vi "PythonNode_testforloopcopy2.vi"() -> ()   [LabVIEW 2023]
doc: "This example demonstrates how to call a Python function and pass doubles as arguments. It uses a python function to compute the sum of two doubles."
uses:
  <vilib>/Utility/sysdir.llb/System Directory Type.ctl
  <vilib>/Utility/file.llb/Write Delimited Spreadsheet (string).vi
panel:
  out "Image":T1(plugin-control)
  out "Waveform Graph":dbl[](graph)
  out "possibility(%)":dbl format="%#_13g"
  out "ready?":string
  out "error out":errorcluster
  in  "error in (no error)":errorcluster
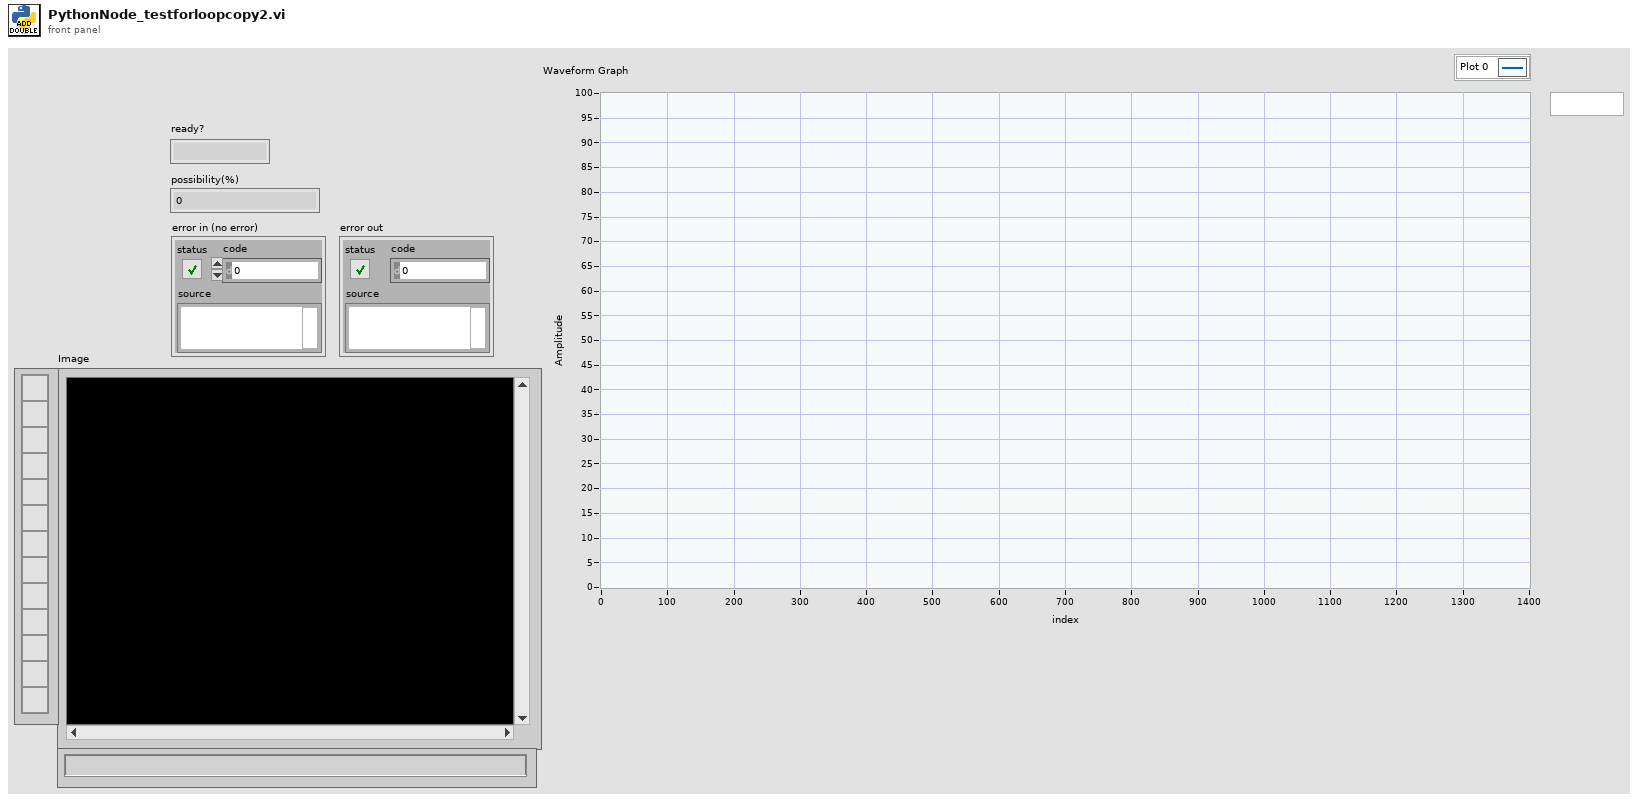
[diagram p1: front panel]
types:
  T1 = typedef "IMAQ Image.ctl" = refnum<image>
  T2 = typedef "System Directory Type.ctl" = i32
  T3 = typedef "Image Type" = u32
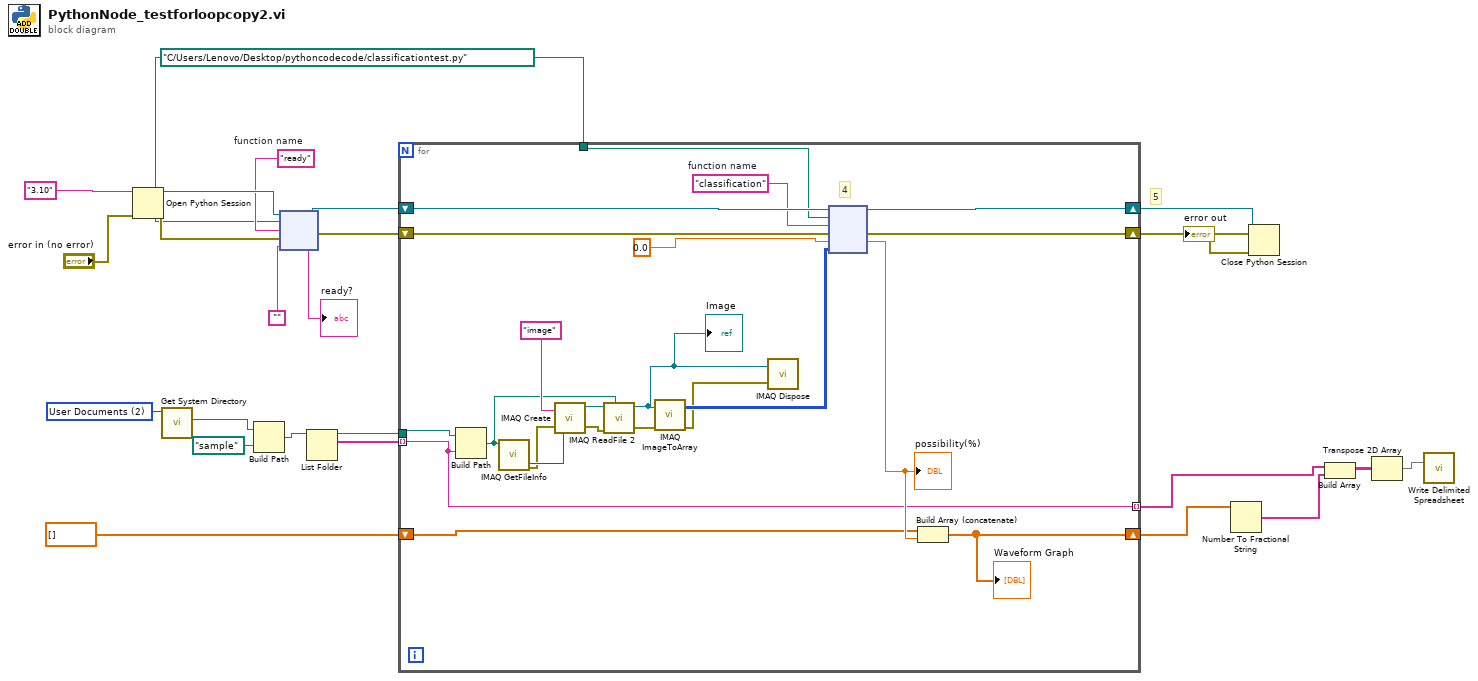
[diagram p0: block diagram]
diagram:
  w12 = T2 2 items=["User Home"=0, "User Desktop"=1, "User Documents"=2, "User Application Data"=3, "User Preferences"=4, "User Temporary"=5, "Public Documents"=6, "Public Application Data"=7, "Public Preferences"=8, "Public Cache"=13, "System Core Libraries"=9, "System Installed Libraries"=10, "Application Files"=11, "Boot Volume Root"=12] ("system directory type")
  w13 = path "C:/Users/Lenovo/Desktop/pythoncodecode/classificationtest.py" ("python file path")
  w21 = "ready"  # function name
  # "5"
  n1 = Open Python Session(python version="3.10", 3:"error in (no error)") -> (session out=w23:refnum<k35>, error out=w22:errorcluster)  [unwired: 1 in]
  n2 = call <vilib>:"Get System Directory.vi"("system directory type"=w12) -> ("system directory"=w11:path)  [unwired: 10 in]
  n3 = Build Path(base path=w11, name or relative path=path "sample") -> (appended path=w9:path)
  n4 = node(w23, w13, w21, w22, "") -> (w19:refnum<k35>, w18:errorcluster, →"ready?":string)  [unwired: 2 out]
  n5 = List Folder(path=w9) -> (path out=w7:path, filenames=w8:string[])  [unwired: 3 in, 2 out]
  n6 = for {
    tunnel: w13 -> [w43]
    shift-right: [w45] -> w17
    shift-left: w19 -> [w47]
    shift-right: [w44] -> w16
    shift-left: w18 -> [w46]
    tunnel: w8 -> [w27] mode=indexing
    tunnel: w7 -> [w36]
    shift-right: [w32] -> w5
    shift-left: dbl[] [] -> [w33]
    tunnel: [w27] -> w4 mode=indexing
    w42 = "classification"  # function name
    # "4"
    n7 = Build Path(base path=w36, name or relative path=w27) -> (appended path=w35:path)
    n8 = call "IMAQ GetFileInfo"("File Path"=w35) -> ("error out"=w28:errorcluster, "Image Type"=w37:T3)  [unwired: 4 in, 5 out]
    n9 = call "IMAQ Create"("Image Name"="image", "Image Type"=w37, "error in (no error)"=w28) -> ("New Image"=w38:T1, "error out"=w29:errorcluster)  [unwired: 2 in]
    n10 = call "IMAQ ReadFile 2"("File Path"=w35, "error in (no error)"=w29, "Image"=w38) -> ("error out"=w30:errorcluster, "Image Out"=w26:T1)  [unwired: 4 in, 3 out]
    "Image" <- w26
    n11 = call "IMAQ ImageToArray"("error in (no error)"=w30, "Image"=w26) -> ("error out"=w31:errorcluster, "Image Pixels (U8)"=w40:u8[][])  [unwired: 2 in, 3 out]
    n12 = call "IMAQ Dispose"("Image"=w26, "error in (no error)"=w31) -> ()  [unwired: 4 in, 1 out]
    n13 = node(w47, w43, w42, w46, 0.0 ("a"), w40) -> (w45:refnum<k35>, w44:errorcluster, w34:dbl)  [unwired: 1 in, 2 out]
    "possibility(%)" <- w34
    n14 = Build Array (concatenate)(w33, w34) -> (w32:dbl[])
    "Waveform Graph" <- w32
  }
  n15 = Number To Fractional String(number=w5) -> (F-format string=w3:string[])  [unwired: 3 in]
  n16 = Close Python Session(session in=w17, error in=w16) -> (11:→"error out":errorcluster)
  n17 = Build Array(w4, w3) -> (w2:string[][])
  n18 = Transpose 2D Array(2D array=w2) -> (transposed array=w1:string[][])
  n19 = call-poly <vilib>:"Write Delimited Spreadsheet.vi"("2D data"=w1) -> ()  [unwired: 13 in, 2 out]
